vi "HomomorphicFilter.vi"(6 "ImgY":i32, 7 "FilterParam":cluster{"D0":u16, "c":dbl, "rl":dbl, "rh":dbl}={"D0"=0, "c"=0.0, "rl"=10.0, "rh"=30.0}, 8 "EorIn":errorcluster, 9 "ImgX":i32) -> (0 "ErrOut":errorcluster, 1 "H(u,v)":dbl[][](array[numeric]))   [LabVIEW 2014]
doc: "Use this template to build a VI to use as a subVI."
panel:
  # "Output Parameters"
  # "Input Parameters"
  # "1) low/high pass filter controlled by D0;\n2) Band pass/reject controlled by D0(low cut) and D1(high cut);\n3) Notch Filter controlled by (+/-u0,+/-v0) and D0;"
  # "VI Description:\nThis VI is .."
  # ":: MVi Framework V1.0 ::\nAuthor:Gaoke Yang\nEmail: gaoke.yang@yahoo.com\nWeb: www.mvicontrol.com\nCopyright (C) 2015, MVI Technologies All Rights Reserved"
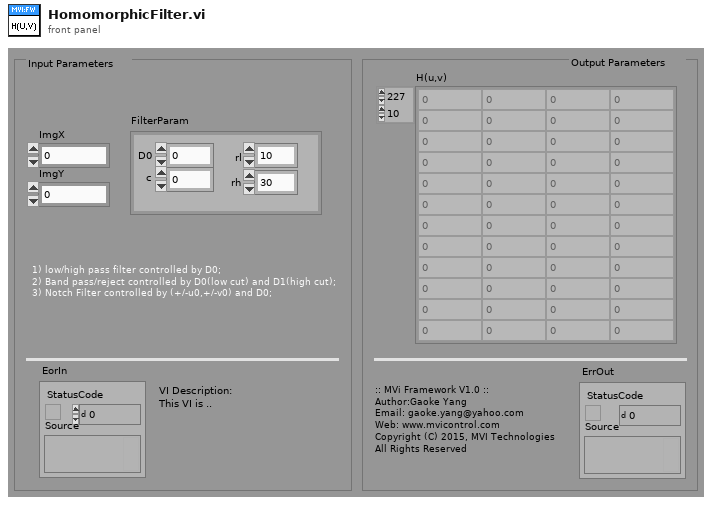
[diagram p1: front panel]
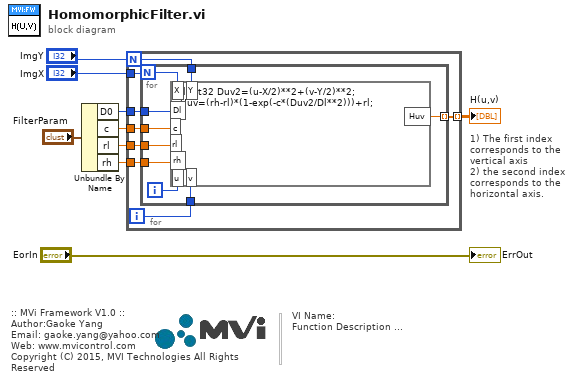
[diagram p0: block diagram]
diagram:
  # "1) The first index corresponds to the vertical axis \n2) the second index corresponds to the horizontal axis."
  # "VI Name:\nFunction Description ..."
  # ":: MVi Framework V1.0 ::\nAuthor:Gaoke Yang\nEmail: gaoke.yang@yahoo.com\nWeb: www.mvicontrol.com\nCopyright (C) 2015, MVI Technologies All Rights Reserved"
  n1 = Unbundle By Name("FilterParam") -> ("D0"=w4:u16, "c"=w3:dbl, "rl"=w2:dbl, "rh"=w1:dbl)
  n2 = for {
    N: "ImgY" -> [w13]
    tunnel: "ImgX" -> [w17]
    tunnel: w4 -> [w16]
    tunnel: w3 -> [w15]
    tunnel: [w12] -> w6 mode=indexing
    tunnel: w2 -> [w11]
    tunnel: w1 -> [w10]
    i -> [w14]
    n3 = for {
      N: w17 -> [w23]
      tunnel: w16 -> [w26]
      tunnel: w15 -> [w20]
      tunnel: w14 -> [w24]
      tunnel: w13 -> [w22]
      tunnel: [w21] -> w12 mode=indexing
      tunnel: w11 -> [w19]
      tunnel: w10 -> [w18]
      i -> [w25]
      n4 = formula code="float32 Duv2=(u-X/2)**2+(v-Y/2)**2;\nHuv=(rh-rl)*(1-exp(-c*(Duv2/Dl**2)))+rl;"("u"=w25, "v"=w24, "Dl"=w26, "Y"=w22, "X"=w23, "c"=w20, "rl"=w19, "rh"=w18) -> ("Huv"=w21:dbl)
    }
  }
  "H(u,v)" <- w6
  "ErrOut" <- "EorIn"
